vi "Warning Log.vi"(10 "Caller":refnum<queue>, 11 "Name":string) -> (2 "Current":string[][](array[string]))   [LabVIEW 2020]
uses:
  02d32eae-ad29-4b14-84d7-b92f461c78f5.vi
  2d64119b-2a62-40b3-aa75-b9f4cd3af465.vi
  01a802db-9668-4dff-9e9f-a0f694c92dc4.vi
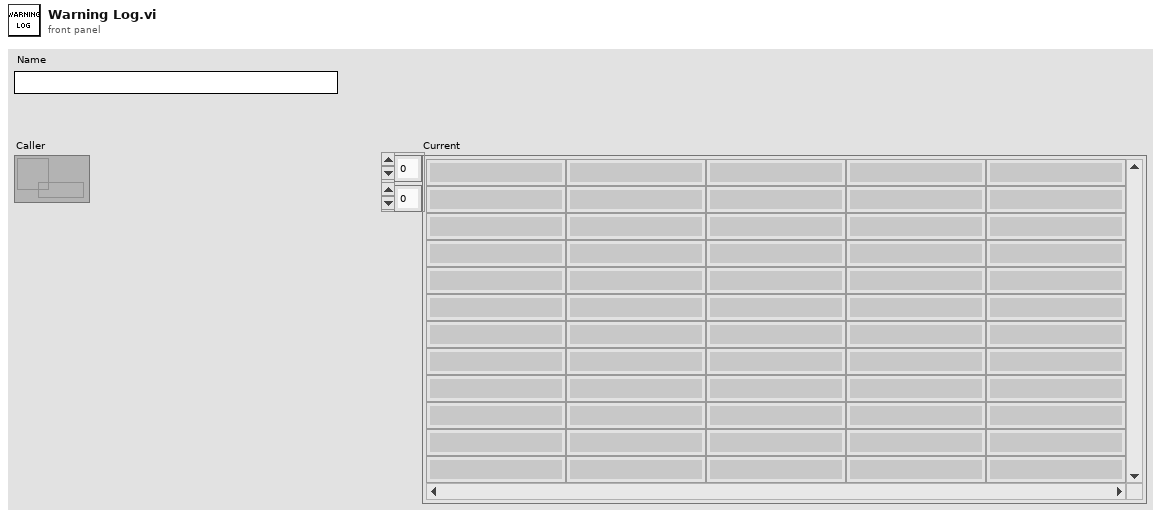
[diagram p1: front panel]
types:
  T1 = typedef "SDQ Data Type.ctl" = cluster{"CAN Length":string, "CAN Name":string, "CAN ID":string, "CAN Type":string, "Test Item":string, "Byte Order":string, "Instruction":string, "Control Type":string, "Group":string, "Offset":dbl, "Coefficient":dbl, "Write Enable":bool, "Lable Type":string, "Key?":string, "Set Value":string, "Upper":dbl, "Lower":dbl, "Unit":string, "Formula":string, "Test Item Type":string, "Length":i32, "Address":string, "Name":string, "Identifier":string, "Data Type":string, "Enumerate?":string, "Enumerate List":string, "Data":string, "Source":string}
  T2 = map{string, cluster{"Warning":string, "level":enum16{"", "Ⅰ", "Ⅱ", "Ⅲ", "Ⅳ", "Ⅴ"}}}
  T3 = map{string, cluster{"Upper Limit":dbl, "Upper Warning":dbl, "Lower Limit":dbl, "Lower Warning":dbl, "level":enum16{"", "Ⅰ", "Ⅱ", "Ⅲ", "Ⅳ", "Ⅴ"}}}
  T4 = cluster{"Warning":string, "level":enum16{"", "Ⅰ", "Ⅱ", "Ⅲ", "Ⅳ", "Ⅴ"}}
  T5 = cluster{"Upper Limit":dbl, "Upper Warning":dbl, "Lower Limit":dbl, "Lower Warning":dbl, "level":enum16{"", "Ⅰ", "Ⅱ", "Ⅲ", "Ⅳ", "Ⅴ"}}
  T6 = cluster{"字符串":string, "level":enum16{"", "Ⅰ", "Ⅱ", "Ⅲ", "Ⅳ", "Ⅴ"}}
  T7 = typedef "SY_Parameter.ctl" = cluster{"RH(%)":cluster{"DS":cluster{"阳极露点温度_DS":string, "阳极出口温度_DS":string, "阴极露点温度_DS":string, "阴极出口温度_DS":string, "阳极相对湿度_DS":string, "阴极相对湿度_DS":string, "阳极露点温度设置_DS":string, "阳极出口温度设置_DS":string, "阴极露点温度设置_DS":string, "阴极出口温度设置_DS":string}, "Value":cluster{"阳极露点温度_PV":sgl, "阳极出口温度_PV":sgl, "阴极露点温度_PV":sgl, "阴极出口温度_PV":sgl, "阳极相对湿度_SY":sgl, "阴极相对湿度_SY":sgl, "阳极露点温度设置_SV":sgl, "阳极出口温度设置_SV":sgl, "阴极露点温度设置_SV":sgl, "阴极出口温度设置_SV":sgl}}, "WEB":cluster{"DS":cluster{"自动模式(M0A1)_DS":string, "设备运行_DS":string, "工步号_DS":string, "运行模式_DS":string}, "Value":cluster{"自动模式(M0A1)_PV":bool, "设备运行_PV":bool, "工步号_PV":sgl, "运行模式_PV":bool}}, "ELD":cluster{"DS":cluster{"负载电压设置_DS":string, "负载电流设置_DS":string, "负载功率设置_DS":string, "负载模式设置_DS":string, "错误代码_DS":string, "负载电压_DS":string, "负载电流_DS":string, "负载功率_DS":string, "负载输出使能_DS":string, "负载连接_DS":string, "负载升压_DS":string, "负载升流_DS":string, "负载升功率_DS":string, "负载降压_DS":string, "负载降流_DS":string, "负载降功率_DS":string, "电流密度_DS":string, "功率密度_DS":string}, "Value":cluster{"负载电压设置_SV":sgl, "负载电流设置_SV":sgl, "负载功率设置_SV":sgl, "负载模式设置_SV":string, "错误代码_PV":string, "负载电压_PV":sgl, "负载电流_PV":sgl, "负载功率_PV":sgl, "负载输出使能_SV":bool, "负载连接_SY":bool, "负载升压_SV":sgl, "负载升流_SV":sgl, "负载升功率_SV":sgl, "负载降压_SV":sgl, "负载降流_SV":sgl, "负载降功率_SV":sgl, "电流密度_SV":sgl, "功率密度_SV":sgl}}, "SY":cluster{"DS":cluster{"总报警_DS":string, "WEB连接_DS":string, "计量比功能_DS":string, "PLC连接_DS":string, "H2计量比功能_DS":string, "Air计量比功能_DS":string, "PLC失联报警_DS":string}, "Value":cluster{"总报警_PV":bool, "WEB连接_PV":bool, "计量比功能_SV":bool, "PLC连接_SV":bool, "H2计量比功能_SV":bool, "Air计量比功能_SV":bool, "PLC失联报警_SV":bool}}, "PLC":cluster{"DS":cluster{"PLC急停_DS":string, "PLC连接_DS":string, "下位机心跳值_DS":string, "上位机心跳值_DS":string, "上位机报警等级字_DS":string, "负载可卸载_DS":string}, "Value":cluster{"PLC急停_PV":bool, "PLC连接_PV":bool, "下位机心跳值_PV":sgl, "上位机心跳值_SV":sgl, "上位机报警等级字_SV":sgl, "负载可卸载_SV":bool}}, "Bool Control":cluster{"DS":cluster{"维护模式_DS":string, "阳极氮气吹扫_DS":string, "阴极氮气吹扫_DS":string, "阳极脉冲使能_DS":string, "准备好使能_DS":string, "阳极干湿气切换_DS":string, "阴极干湿气切换_DS":string, "自动/手动模式_DS":string, "入口背压_DS":string, "手动卸载_DS":string, "软急停_DS":string, "负载连接_DS":string, "PLC故障复位_DS":string, "蜂鸣器屏蔽_DS":string}, "Value":cluster{"维护模式_SV":bool, "阳极氮气吹扫_SV":bool, "阴极氮气吹扫_SV":bool, "阳极脉冲使能_SV":bool, "准备好使能_SV":bool, "阳极干湿气切换_SV":bool, "阴极干湿气切换_SV":bool, "自动/手动模式_SV":bool, "入口背压_SV":bool, "手动卸载_SV":bool, "软急停_SV":bool, "负载连接_SV":bool, "PLC故障复位_SV":bool, "蜂鸣器屏蔽_SV":bool}}, "Stoich":cluster{"DS":cluster{"H2初始流量_DS":string, "Ait初始流量_DS":string, "H2侧系数_DS":string, "Air侧系数_DS":string, "H2计量比_DS":string, "Air计量比_DS":string, "时间间隔_DS":string, "H2计算气量_DS":string, "Air计算气量_DS":string, "H2流量_DS":string, "Air流量_DS":string}, "Value":cluster{"H2初始流量_SV":sgl, "Ait初始流量_SV":sgl, "H2侧系数_SV":sgl, "Air侧系数_SV":sgl, "H2计量比_SV":sgl, "Air计量比_SV":sgl, "时间间隔_SV":sgl, "H2计算气量_SV":sgl, "Air计算气量_SV":sgl, "H2流量_DS":sgl, "Air流量_DS":sgl}}, "PLC Need":cluster{"Name":string, "Identifier":string, "Source":string, "Value":string}[], "CVM":cluster{"DS":cluster{"活化面积_DS":string, "开路电压_DS":string, "单体总片数_DS":string, "单体显示片数_DS":string, "起始编号_DS":string, "最大值":string, "最大值编号_DS":string, "最小值_DS":string, "最小值编号_DS":string, "选区合计电压_DS":string, "平均值_DS":string, "离均差_DS":string}, "Value":cluster{"活化面积_SV":sgl, "开路电压_SV":sgl, "单体片数_SV":sgl, "单体显示片数_SV":sgl, "起始编号_SV":sgl, "最大值_SV":sgl, "最大值编号_SV":sgl, "最小值_SV":sgl, "最小值编号_SV":sgl, "选区合计电压_SV":sgl, "平均值_SV":sgl, "离均差_SV":sgl}}}
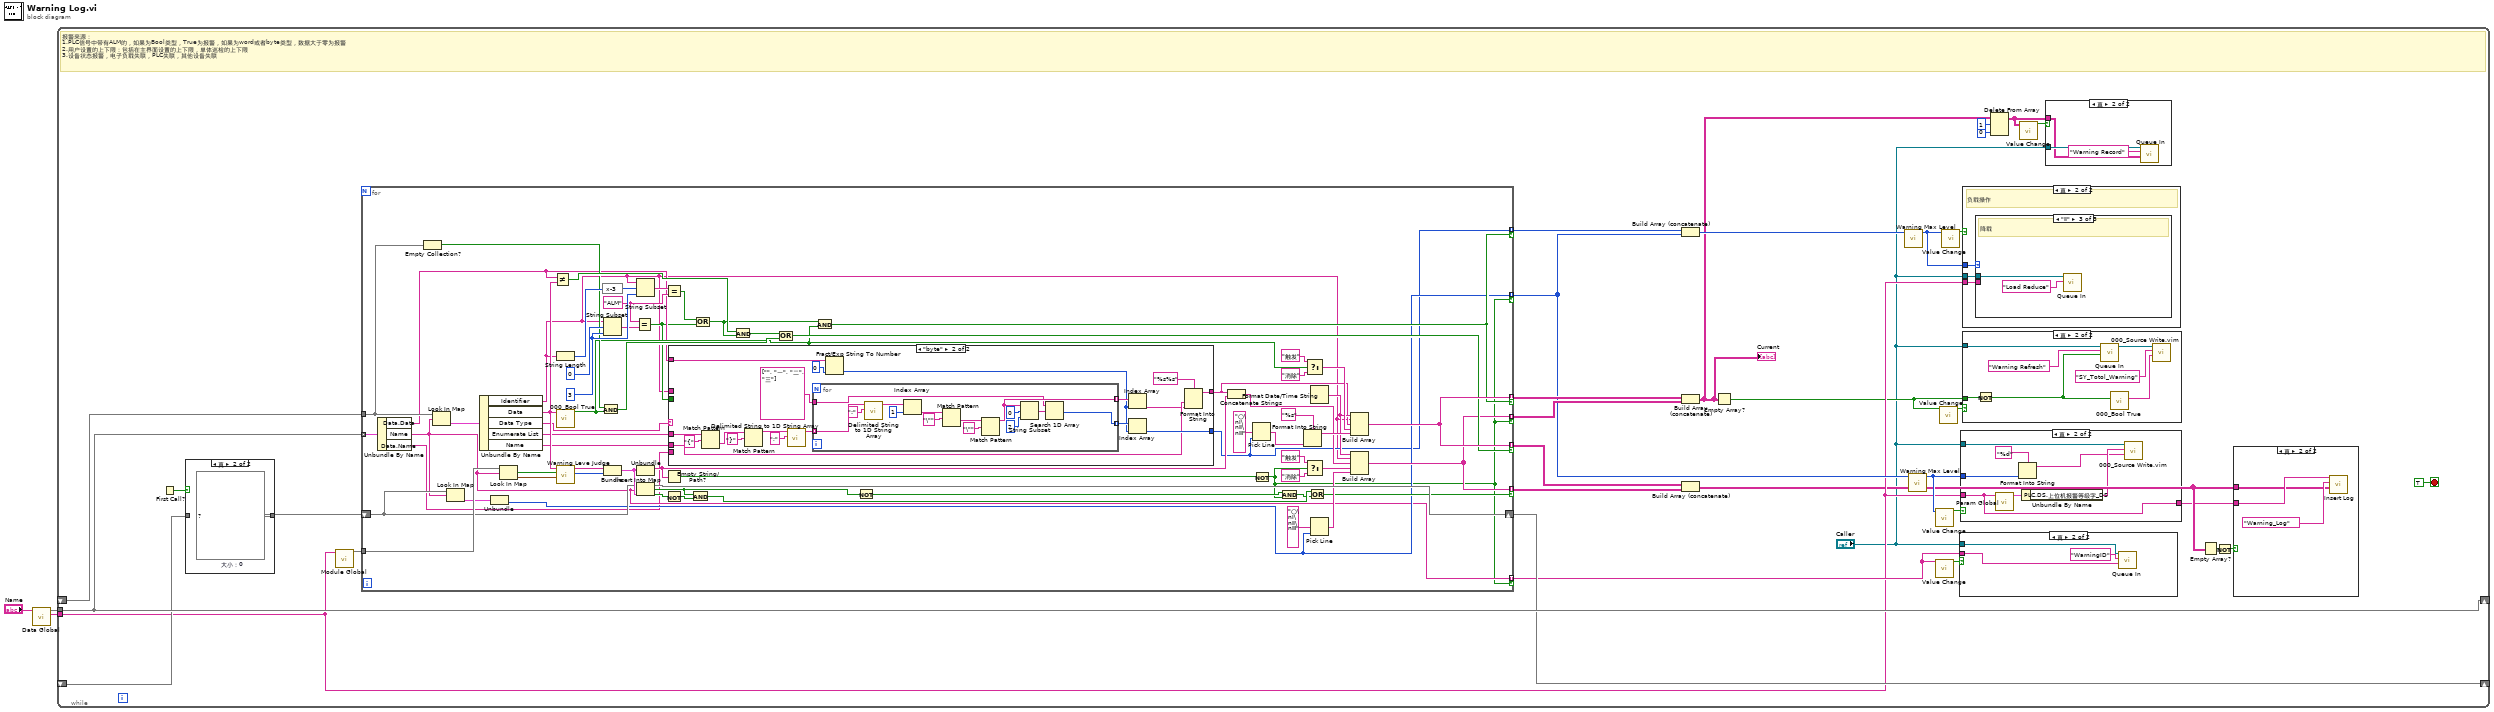
[diagram p0: block diagram]
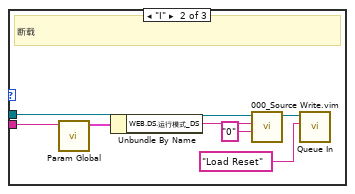
[diagram p9: hidden frame]
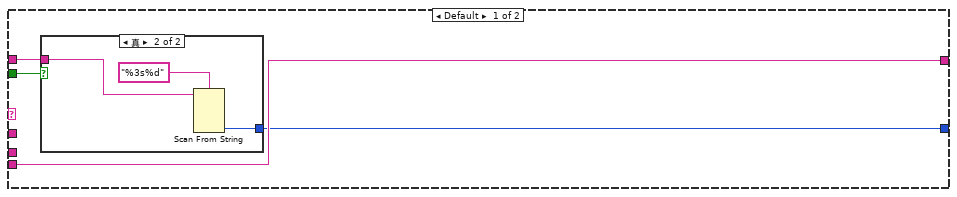
[diagram p11: hidden frame]
diagram:
  n1 = call "Data Global.vi"("Name"="Name") -> ("Project"=w1:string, "Data Out"=w3:map{string, T1})  [unwired: 7 in, 2 out]
  n2 = while {
    shift-right: [w35] -> _
    shift-left: _ -> [w37]
    tunnel: w3 -> [w35]
    tunnel: w1 -> [w17]
    shift-right: [w32] -> _
    shift-left: _ -> [w31]
    stop <- TRUE stop-if-true
    # "报警来源：\n1.PLC信号中带有ALM的，如果为Bool类型，True为报警，如果为word或者byte类型，数据大于零为报警\n2.用户设置的上下限：包括在主界面设置的上下限，单体巡检的上下限\n3.设备状态报警，电子负载失联，PLC失联，其他设备失联"
    n3 = First Call?() -> (First Call?: T/F=w24:bool)
    n4 = case shown="真" w24 {
      tunnel: [w74 w75] -> w33
      tunnel: w31 -> [w74 _]
      frame False {
      }
      frame True {
        w75 = T2 {}  # 大小：0
      }
    }
    n5 = call "Module Global.vi"("Project"=w17) -> ("Limit Out"=w34:T3)  [unwired: 9 in, 1 out]
    n6 = for {
      tunnel: w37 -> [w123]
      tunnel: w35 -> [w118] mode=indexing
      tunnel: [w124] -> w30 mode=indexing if=w119
      tunnel: [w124] -> w28 mode=indexing if=w89
      tunnel: w34 -> [w115]
      shift-right: [w112] -> w32
      shift-left: w33 -> [w102]
      tunnel: [w93] -> w27 mode=indexing if=w86
      tunnel: [w93] -> w29 mode=indexing if=w92
      tunnel: [w81] -> w26 mode=indexing if=w89
      tunnel: [w88] -> w25 mode=indexing if=w86
      tunnel: [w87] -> w19 mode=indexing if=w86
      w136 = "ALM" ("正则表达式")
      w141 = 3 ("长度（剩余）")
      n7 = Unbundle By Name(w118) -> ("Data.Data"=w84:string, "Name"=w87:string, "Data.Name"=w83:string)
      n8 = Empty Collection?(1:w123) -> (0:w122:bool)
      n9 = Look In Map(map=w123, key=w87) -> (value=w133:T1)  [unwired: 1 in, 1 out]
      n10 = Look In Map(map=w102, key=w87) -> (value=w101:T4)  [unwired: 1 in, 1 out]
      n11 = Unbundle By Name(w133) -> ("Identifier"=w79:string, "Data"=w85:string, "Data Type"=w78:string, "Enumerate List"=w77:string, "Name"=w76:string)
      n12 = Unbundle(w101) -> ("level"=w88:enum16{"", "Ⅰ", "Ⅱ", "Ⅲ", "Ⅳ", "Ⅴ"})  [unwired: 1 out]
      n13 = Look In Map(map=w115, key=w87) -> (key not found?=w113:bool, value=w114:T5)  [unwired: 1 in]
      n14 = Not Equal?(x=w84, y=w85) -> (x != y?=w126:bool)
      n15 = String Length(string=w79) -> (length=w139:i32)
      n16 = call "000_Bool True.vi"("Bool String"=w85) -> ("True"=w117:bool)  [unwired: 8 in, 2 out]
      n17 = call "Warning Leve Judge.vi"("Limit"=w114, "key not found?"=w113, "Data"=w85) -> ("level"=w110:enum16{"", "Ⅰ", "Ⅱ", "Ⅲ", "Ⅳ", "Ⅴ"}, "字符串"=w111:string)  [unwired: 7 in]
      n18 = expression code="x-3"(w139) -> (w140:i32)
      n19 = And(x=w122, y=w117) -> (x .and. y?=w120:bool)
      n20 = String Subset(string=w79, offset (0)=0 ("偏移量(0)"), length (rest)=w141) -> (substring=w135:string)
      n21 = Bundle("字符串"=w111, "level"=w110) -> (w105:T6)  [unwired: 1 in]
      n22 = Equal?(x=w136, y=w135) -> (x = y?=w80:bool)
      n23 = String Subset(string=w79, offset (0)=w140, length (rest)=w141) -> (substring=w137:string)
      n24 = Unbundle(w105) -> ("字符串"=w91:string)  [unwired: 1 out]
      n25 = Insert Into Map(map in=w102, key=w87, value=w105) -> (map out=w112:T2, key already included?=w106:bool, value unchanged?=w109:bool)
      n26 = Equal?(x=w137, y=w136) -> (x = y?=w134:bool)
      n27 = Empty String/Path?(string/path=w91) -> (empty?=w100:bool)
      n28 = Not(x=w109) -> (.not. x?=w108:bool)
      n29 = case shown="\"byte\"" w78 {
        tunnel: w77 -> [_ w159]
        tunnel: w84 -> [_ w157]
        tunnel: [w142 w153] -> w81
        tunnel: [w145 w149] -> w82
        tunnel: w83 -> [w145 _]
        tunnel: w80 -> [w144 _]
        tunnel: w79 -> [w143 _]
        tunnel: w76 -> [_ w151]
        frame Default {
          n30 = case shown="真" w144 {
            tunnel: w143 -> [_ w147]
            tunnel: [_ w146] -> w142
            frame False {
            }
            frame True {
              n31 = Scan From String(format string="%3s%d" ("格式字符串"), input string=w147) -> (output 2=w146:i32)  [unwired: 5 in, 3 out]
            }
          }
        }
        frame "byte" {
          n32 = Match Pattern(string=w159, regular expression="{" ("正则表达式")) -> (after substring=w165:string)  [unwired: 1 in, 3 out]
          n33 = Match Pattern(string=w165, regular expression="}" ("正则表达式")) -> (before substring=w163:string)  [unwired: 1 in, 3 out]
          n34 = call <vilib>:"Delimited String to 1D String Array.vi"("delimiter"=";", "delimited string"=w163) -> ("string array"=w161:string[])  [unwired: 9 in]
          n35 = for {
            tunnel: w161 -> [w179] mode=indexing
            tunnel: [w172] -> w158 mode=indexing
            tunnel: string[] ["", "一", "二", "三"] -> [w169]
            tunnel: [w167] -> w156 mode=indexing
            n36 = call <vilib>:"Delimited String to 1D String Array.vi"("delimiter"=":", "delimited string"=w179) -> ("string array"=w175:string[])  [unwired: 9 in]
            n37 = Index Array(array=w175, index=1 ("索引")) -> (element=w173:string)
            n38 = Match Pattern(string=w173, regular expression="\"" ("正则表达式")) -> (after substring=w177:string)  [unwired: 1 in, 3 out]
            n39 = Match Pattern(string=w177, regular expression="\"" ("正则表达式")) -> (before substring=w172:string)  [unwired: 1 in, 3 out]
            n40 = String Subset(string=w172, offset (0)=0 ("偏移量(0)"), length (rest)=2 ("长度（剩余）")) -> (substring=w168:string)
            n41 = Search 1D Array(1D array=w169, element=w168) -> (index of element=w167:i32)  [unwired: 1 in]
          }
          n42 = Fract/Exp String To Number(string=w157, default (0 dbl)=u32 0 ("默认(0 DBL)")) -> (number=w155:u32)  [unwired: 2 in, 1 out]
          n43 = Index Array(array=w158, index=w155) -> (element=w150:string)
          n44 = Index Array(array=w156, index=w155) -> (element=w153:i32)
          n45 = Format Into String(format string="%s%s" ("格式字符串"), w151, w150) -> (resulting string=w149:string)  [unwired: 2 in, 1 out]
        }
      }
      n46 = And(x=w106, y=w108) -> (x .and. y?=w107:bool)
      n47 = Compound Arithmetic op=OR ("复合运算")(w134, w80) -> (w116:bool)
      n48 = And(x=w126, y=w116) -> (x .and. y?=w121:bool)
      n49 = Compound Arithmetic op=OR ("复合运算")(w121, w120) -> (w119:bool)
      n50 = And(x=w116, y=w117) -> (x .and. y?=w89:bool)
      n51 = Not(x=w106) -> (.not. x?=w104:bool)
      n52 = Concatenate Strings(w82, w91) -> (w90:string)
      n53 = Pick Line(multi-line string="〇\nⅠ\nⅡ\nⅢ", line index=w81) -> (output string=w129:string)  [unwired: 1 in]
      n54 = Not(x=w100) -> (.not. x?=w86:bool)
      n55 = And(x=w104, y=w86) -> (x .and. y?=w103:bool)
      n56 = Format Into String(format string="%s" ("格式字符串"), w129) -> (resulting string=w128:string)  [unwired: 2 in, 1 out]
      n57 = Select(t="触发" ("ON"), s=w117, f="消除" ("OFF")) -> (s? t:f=w127:string)
      n58 = Select(t="触发" ("ON"), s=w86, f="消除" ("OFF")) -> (s? t:f=w96:string)
      n59 = Or(x=w107, y=w103) -> (x .or. y?=w92:bool)
      n60 = Pick Line(multi-line string="〇\nⅠ\nⅡ\nⅢ", line index=w88) -> (output string=w94:string)  [unwired: 1 in]
      n61 = Format Date/Time String() -> (date/time string=w99:string)  [unwired: 3 in]
      n62 = Build Array(w99, w79, w82, w127, w128) -> (w124:string[])
      n63 = Build Array(w99, w79, w90, w96, w94) -> (w93:string[])
    }
    n64 = Build Array (concatenate)(w26, w25) -> (w12:i32[])
    n65 = Build Array (concatenate)(w28, w27) -> (w9:string[][])
    "Current" <- w9
    n66 = Build Array (concatenate)(w30, w29) -> (w14:string[][])
    n67 = Empty Array?(array=w9) -> (empty?=w10:bool)
    n68 = call "Warning Max Level.vi"("数组"=w12) -> ("level"=w11:enum16{"", "Ⅰ", "Ⅱ", "Ⅲ", "Ⅳ", "Ⅴ"})  [unwired: 10 in]
    n69 = call "Warning Max Level.vi"("数组"=w25) -> ("level"=w22:enum16{"", "Ⅰ", "Ⅱ", "Ⅲ", "Ⅳ", "Ⅴ"})  [unwired: 10 in]
    n70 = call "Value Change.vi"("New Data"=w22) -> ("Change?"=w21:bool)  [unwired: 10 in]
    n71 = call "Value Change.vi"("New Data"=w19) -> ("Change?"=w20:bool)  [unwired: 10 in]
    n72 = call "Value Change.vi"("New Data"=w10) -> ("Change?"=w18:bool)  [unwired: 10 in]
    n73 = call "Value Change.vi"("New Data"=w11) -> ("Change?"=w23:bool)  [unwired: 10 in]
    n74 = case shown="真" w20 {
      tunnel: "Caller" -> [_ w52]
      tunnel: w19 -> [_ w51]
      frame False {
      }
      frame True {
        n75 = call "Queue In.vi"("Data"=w51, "Message"="WarningID", "Queue In"=w52) -> ()  [unwired: 7 in, 2 out]
      }
    }
    n76 = case shown="真" w21 {
      tunnel: w22 -> [_ w60]
      tunnel: w17 -> [w54 w55]
      tunnel: "Caller" -> [_ w58]
      tunnel: [w54 w55] -> w13
      frame False {
      }
      frame True {
        n77 = call "Param Global.vi"("Project"=w55) -> ("Param Out"=w59:T7)  [unwired: 9 in, 1 out]
        n78 = Format Into String(format string="%d" ("格式字符串"), w60) -> (resulting string=w56:string)  [unwired: 2 in, 1 out]
        n79 = Unbundle By Name(w59) -> ("PLC.DS.上位机报警等级字_DS"=w57:string)
        n80 = call "000_Source Write.vim"("Data"=w56, "Name"=w57, "Queue In"=w58) -> ()  [unwired: 6 in, 3 out]
      }
    }
    n81 = case shown="真" w23 {
      tunnel: w11 -> [_ w64]
      tunnel: "Caller" -> [_ w63]
      tunnel: w17 -> [_ w62]
      frame False {
      }
      frame True {
        # "负载操作"
        n82 = case shown="\"Ⅱ\"" w64 {
          tunnel: w63 -> [_ w71 w73]
          tunnel: w62 -> [_ w67 _]
          frame Default {
          }
          frame "Ⅰ" {
            # "断载"
            n83 = call "Param Global.vi"("Project"=w67) -> ("Param Out"=w70:T7)  [unwired: 9 in, 1 out]
            n84 = Unbundle By Name(w70) -> ("WEB.DS.运行模式_DS"=w69:string)
            n85 = call "000_Source Write.vim"("Data"="0", "Name"=w69, "Queue In"=w71) -> ("Queue Out"=w66:refnum<queue>)  [unwired: 6 in, 2 out]
            n86 = call "Queue In.vi"("Message"="Load Reset", "Queue In"=w66) -> ()  [unwired: 8 in, 2 out]
          }
          frame "Ⅱ" {
            # "降载"
            n87 = call "Queue In.vi"("Message"="Load Reduce", "Queue In"=w73) -> ()  [unwired: 8 in, 2 out]
          }
        }
      }
    }
    n88 = case shown="真" w18 {
      tunnel: "Caller" -> [_ w50]
      tunnel: w10 -> [_ w45]
      frame False {
      }
      frame True {
        n89 = Not(x=w45) -> (.not. x?=w44:bool)
        n90 = call "Queue In.vi"("Data"=w44, "Message"="Warning Refresh", "Queue In"=w50) -> ("Queue Out"=w48:refnum<queue>)  [unwired: 7 in, 1 out]
        n91 = call "000_Bool True.vi"("Value"=w44) -> ("String Out"=w46:string)  [unwired: 8 in, 2 out]
        n92 = call "000_Source Write.vim"("Data"=w46, "Name"="SY_Totol_Warning", "Queue In"=w48) -> ()  [unwired: 6 in, 3 out]
      }
    }
    n93 = Delete From Array(array=w9, length=1 ("长度"), index (col)=0 ("禁用的索引 (列)")) -> (array with subset deleted=w6:string[][])  [unwired: 1 in, 1 out]
    n94 = call "Value Change.vi"("New Data"=w6) -> ("Change?"=w7:bool)  [unwired: 10 in]
    n95 = case shown="真" w7 {
      tunnel: "Caller" -> [_ w40]
      tunnel: w6 -> [_ w39]
      frame False {
      }
      frame True {
        n96 = call "Queue In.vi"("Data"=w39, "Message"="Warning Record", "Queue In"=w40) -> ()  [unwired: 7 in, 2 out]
      }
    }
    n97 = Empty Array?(array=w14) -> (empty?=w16:bool)
    n98 = Not(x=w16) -> (.not. x?=w15:bool)
    n99 = case shown="真" w15 {
      tunnel: w13 -> [_ w42]
      tunnel: w14 -> [_ w41]
      frame False {
      }
      frame True {
        n100 = call "Insert Log.vi"("Data"=w41, "Table"="Warning_Log", "Project"=w42) -> ()  [unwired: 8 in, 1 out]
      }
    }
  }
